vi "Fabry-Peort-dV_tune-to_T1_T2.vi"() -> ()   [LabVIEW 2010]
panel:
  in  "Fudge 1":dbl=1.14 format="%_6g"
  in  "Fudge 2":dbl=1.035 format="%_6g"
  out "Et 2 T(K)  to":dbl=101.5201705599927
  out "Temperature orders Et2":dbl[](array[numeric])=[62.87717711991215, 101.5201705599927, 127.00507430677763, 148.86661269772853, 167.98956620502332, 185.12165410677824] format="%.2f"
  in  "Et 2 T(K)  initial":dbl=58.52
  in  "Et 2 thickness at 300K":dbl=250.0 format="%.1f"
  out "Temperature orders Et1":dbl[](array[numeric])=[73.33983498145668, 112.27280779006229, 140.17409965395515, 163.98820334481977, 184.6134959181669, 203.93828252389144] format="%.2f"
  out "Et 1 T(K)  to":dbl=112.27280779006229
  in  "dV change":dbl=300.0 format="%_6g"
  in  "Wavelength":dbl=1.28 format="%_6g"
  in  "Et 1 thickness at 300K":dbl=210.0 format="%.1f"
  in  "Et 1 T(K)  initial":dbl=78.5
  # "fudge  2 - 1.03500"
  # "fudge  1 - 1.12000"
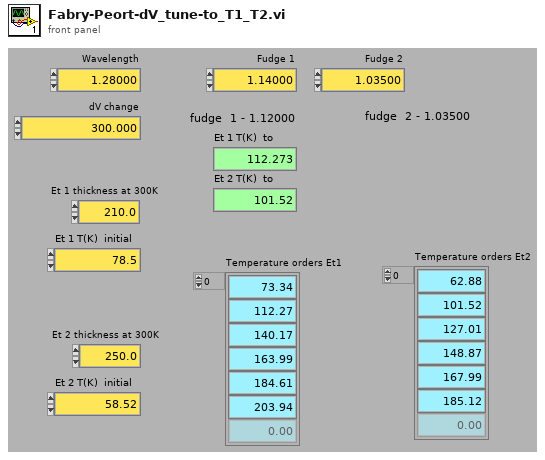
[diagram p1: front panel]
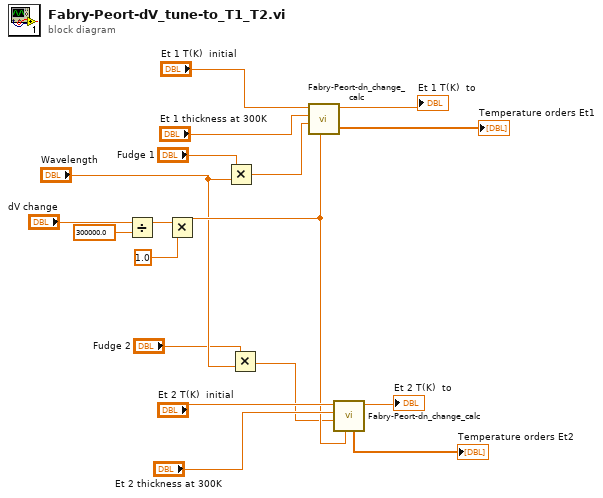
[diagram p0: block diagram]
diagram:
  n1 = Divide(x="dV change", y=300000.0) -> (x/y=w10:dbl)
  n2 = Multiply(x=w10, y=1.0) -> (x*y=w7:dbl)
  n3 = Multiply(x="Fudge 1", y="Wavelength") -> (x*y=w2:dbl)
  n4 = Multiply(x="Fudge 2", y="Wavelength") -> (x*y=w5:dbl)
  n5 = call "Fabry-Peort-dn_change_calc.vi"("dLam chnage"=w7, "Wavelength"=w2, "Et thickness at 300K"="Et 1 thickness at 300K", "Et T(K)  initial"="Et 1 T(K)  initial") -> ("Et T(K)  to"=→"Et 1 T(K)  to":dbl, "Temperature orders Et1 2"=→"Temperature orders Et1":dbl[])  [unwired: 3 in, 3 out]
  n6 = call "Fabry-Peort-dn_change_calc.vi"("dLam chnage"=w7, "Wavelength"=w5, "Et thickness at 300K"="Et 2 thickness at 300K", "Et T(K)  initial"="Et 2 T(K)  initial") -> ("Et T(K)  to"=→"Et 2 T(K)  to":dbl, "Temperature orders Et1 2"=→"Temperature orders Et2":dbl[])  [unwired: 3 in, 3 out]
